vi "set_state.vi"(0 "boolean_indicator_refnum":refnum<vi>, 1 "state_triggers":T1) -> ()   [LabVIEW 2019]
uses:
  state_triggers.ctl
  FGV_DOCK_multistate_indicator_state.ctl
  _misc/AULocalize/SubVIs/Get Localized Phrase Compact Interface 1D.vi
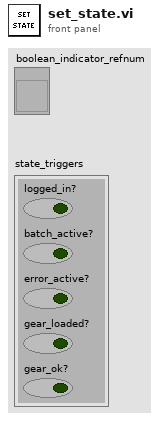
[diagram p1: front panel]
types:
  T1 = typedef "state_triggers.ctl" = cluster{"logged_in?":bool, "batch_active?":bool, "error_active?":bool, "gear_loaded?":bool, "gear_ok?":bool}
  T2 = typedef "FGV_DOCK_multistate_indicator_state.ctl" = enum16{"ready", "gear_OK", "batch_not_started", "logged_out", "gear_NOK", "error"}
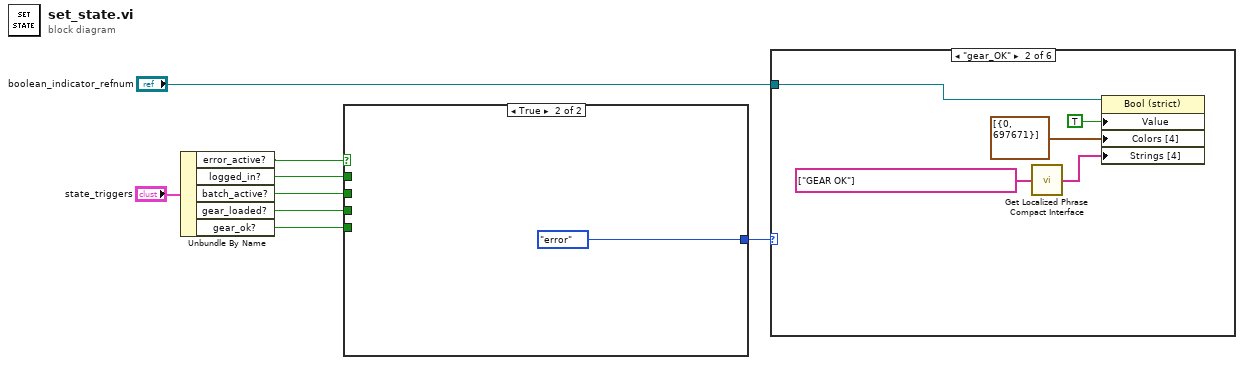
[diagram p0: block diagram]
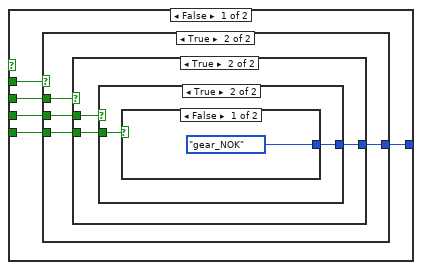
[diagram p2: hidden frame]
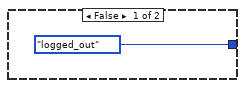
[diagram p3: hidden frame]
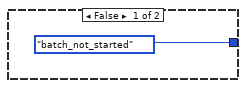
[diagram p4: hidden frame]
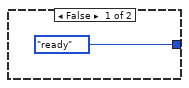
[diagram p5: hidden frame]
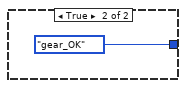
[diagram p6: hidden frame]
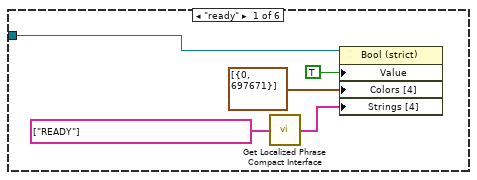
[diagram p7: hidden frame]
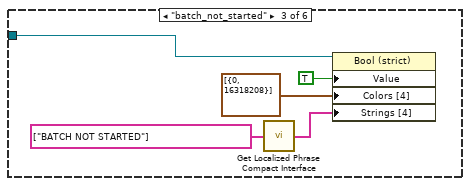
[diagram p8: hidden frame]
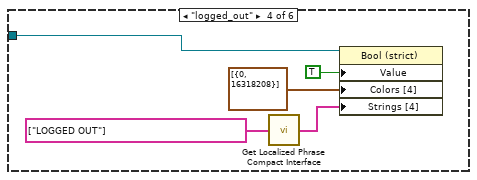
[diagram p9: hidden frame]
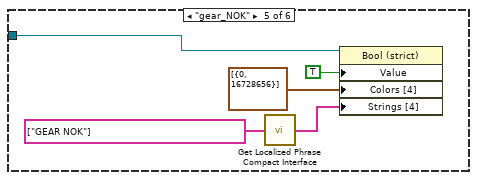
[diagram p10: hidden frame]
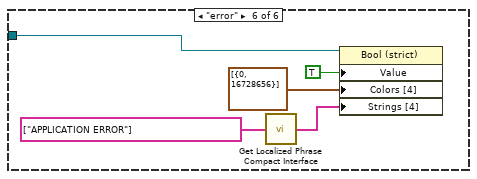
[diagram p11: hidden frame]
diagram:
  n1 = Unbundle By Name("state_triggers") -> ("error_active?"=w5:bool, "logged_in?"=w4:bool, "batch_active?"=w3:bool, "gear_loaded?"=w2:bool, "gear_ok?"=w1:bool)
  n2 = case shown="True" w5 {
    tunnel: [w11 FGV_DOCK_multistate_indicator_state."error" ("state")] -> w7
    tunnel: w4 -> [w13 _]
    tunnel: w3 -> [w12 _]
    tunnel: w2 -> [w10 _]
    tunnel: w1 -> [w9 _]
    frame False {
      n3 = case shown="True" w13 {
        tunnel: w12 -> [_ w18]
        tunnel: [FGV_DOCK_multistate_indicator_state."logged_out" ("state") w17] -> w11
        tunnel: w10 -> [_ w16]
        tunnel: w9 -> [_ w15]
        frame False {
        }
        frame True {
          n4 = case shown="True" w18 {
            tunnel: [FGV_DOCK_multistate_indicator_state."batch_not_started" ("state") w20] -> w17
            tunnel: w16 -> [_ w22]
            tunnel: w15 -> [_ w21]
            frame False {
            }
            frame True {
              n5 = case shown="True" w22 {
                tunnel: w21 -> [_ w25]
                tunnel: [FGV_DOCK_multistate_indicator_state."ready" ("state") w24] -> w20
                frame False {
                }
                frame True {
                  n6 = case shown="False" w25 {
                    tunnel: [FGV_DOCK_multistate_indicator_state."gear_NOK" ("state") FGV_DOCK_multistate_indicator_state."gear_OK" ("state")] -> w24
                    frame False {
                    }
                    frame True {
                    }
                  }
                }
              }
            }
          }
        }
      }
    }
    frame True {
    }
  }
  n7 = case shown="\"gear_OK\"" w7 {
    tunnel: "boolean_indicator_refnum" -> [w33 w38 w43 w48 w53 w58]
    frame "ready" {
      n8 = call-poly "Get Localized Phrase Compact Interface.vi"("Key"=string[] ["READY"] ("Strings [4]")) -> ("Translated Phrase"=w29:string[])
      n9 = property on="Property Node" class="Bool (strict)"(reference=w33, "Value"=TRUE ("Boolean"), "Colors [4]"=cluster{u32, u32}[] [{0, 697671}], "Strings [4]"=w29) -> ()  [unwired: 1 in, 2 out]
    }
    frame "gear_OK" {
      n10 = call-poly "Get Localized Phrase Compact Interface.vi"("Key"=string[] ["GEAR OK"] ("Strings [4]")) -> ("Translated Phrase"=w34:string[])
      n11 = property on="Property Node" class="Bool (strict)"(reference=w38, "Value"=TRUE ("Boolean"), "Colors [4]"=cluster{u32, u32}[] [{0, 697671}], "Strings [4]"=w34) -> ()  [unwired: 1 in, 2 out]
    }
    frame "batch_not_started" {
      n12 = call-poly "Get Localized Phrase Compact Interface.vi"("Key"=string[] ["BATCH NOT STARTED"] ("Strings [4]")) -> ("Translated Phrase"=w39:string[])
      n13 = property on="Property Node" class="Bool (strict)"(reference=w43, "Value"=TRUE ("Boolean"), "Colors [4]"=cluster{u32, u32}[] [{0, 16318208}], "Strings [4]"=w39) -> ()  [unwired: 1 in, 2 out]
    }
    frame "logged_out" {
      n14 = call-poly "Get Localized Phrase Compact Interface.vi"("Key"=string[] ["LOGGED OUT"] ("Strings [4]")) -> ("Translated Phrase"=w44:string[])
      n15 = property on="Property Node" class="Bool (strict)"(reference=w48, "Value"=TRUE ("Boolean"), "Colors [4]"=cluster{u32, u32}[] [{0, 16318208}], "Strings [4]"=w44) -> ()  [unwired: 1 in, 2 out]
    }
    frame "gear_NOK" {
      n16 = call-poly "Get Localized Phrase Compact Interface.vi"("Key"=string[] ["GEAR NOK"] ("Strings [4]")) -> ("Translated Phrase"=w49:string[])
      n17 = property on="Property Node" class="Bool (strict)"(reference=w53, "Value"=TRUE ("Boolean"), "Colors [4]"=cluster{u32, u32}[] [{0, 16728656}], "Strings [4]"=w49) -> ()  [unwired: 1 in, 2 out]
    }
    frame "error" {
      n18 = call-poly "Get Localized Phrase Compact Interface.vi"("Key"=string[] ["APPLICATION ERROR"] ("Strings [4]")) -> ("Translated Phrase"=w54:string[])
      n19 = property on="Property Node" class="Bool (strict)"(reference=w58, "Value"=TRUE ("Boolean"), "Colors [4]"=cluster{u32, u32}[] [{0, 16728656}], "Strings [4]"=w54) -> ()  [unwired: 1 in, 2 out]
    }
  }
